vi "Gallons Adjustment.vi"(6 "Enable?":bool, 9 "Gallon Adder Input":dbl, 10 "Previous Totalizer (Gallons)":dbl, 11 "Current Totalizer (Gallons)":dbl) -> (1 "Gallon Adder Output":dbl, 3 "Normalized Gallons":dbl)   [LabVIEW 2020]
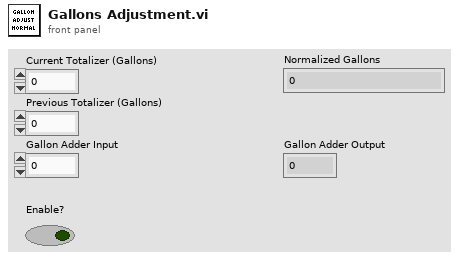
[diagram p1: front panel]
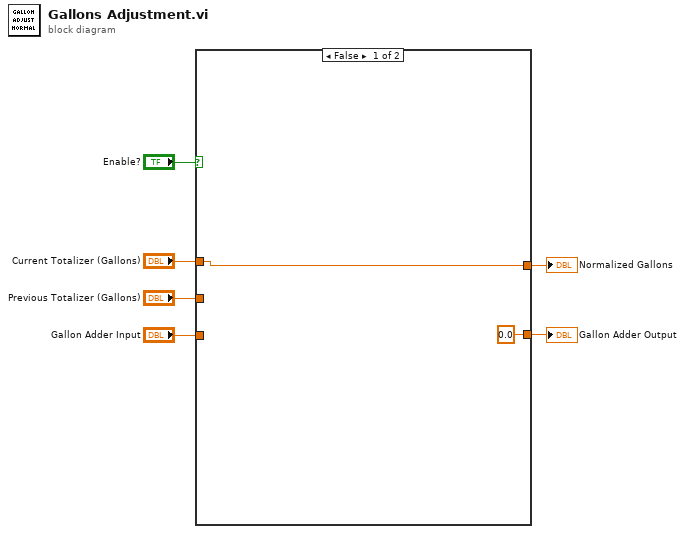
[diagram p0: block diagram]
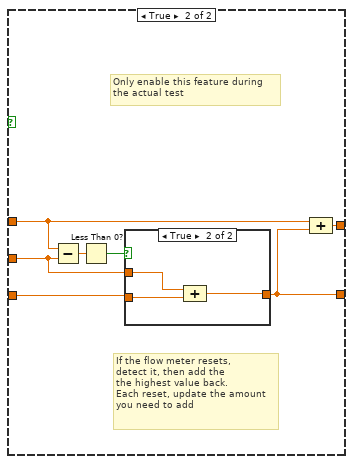
[diagram p2: hidden frame]
diagram:
  n1 = case shown="False" "Enable?" {
    tunnel: "Current Totalizer (Gallons)" -> [w8 w15]
    tunnel: [0.0 ("Gallon Adder Input") w14] -> w5
    tunnel: [w8 w13] -> w4
    tunnel: "Previous Totalizer (Gallons)" -> [_ w11]
    tunnel: "Gallon Adder Input" -> [_ w9]
    frame False {
    }
    frame True {
      # "Only enable this feature during \nthe actual test"
      # "If the flow meter resets,\ndetect it, then add the \nthe highest value back.\nEach reset, update the amount\nyou need to add"
      n2 = Subtract(x=w15, y=w11) -> (x-y=w10:dbl)
      n3 = Less Than 0?(x=w10) -> (x < 0?=w12:bool)
      n4 = case shown="True" w12 {
        tunnel: w9 -> [w16 w19]
        tunnel: [w16 w18] -> w14
        tunnel: w11 -> [_ w17]
        frame False {
        }
        frame True {
          n5 = Compound Arithmetic op=ADD(w17, w19) -> (w18:dbl)
        }
      }
      n6 = Compound Arithmetic op=ADD(w15, w14) -> (w13:dbl)
    }
  }
  "Normalized Gallons" <- w4
  "Gallon Adder Output" <- w5
